vi "Get Element At (Dimensions).vi"(8 "error in (no error)":errorcluster, 10 "Index":i32[](array[numeric]), 11 "Array in":refnum<class "Array.lvclass">) -> (0 "error out":errorcluster, 2 "Element out":refnum<class "Data.lvclass">, 3 "Array out":refnum<class "Array.lvclass">)   [LabVIEW 2012, in "MDSplus.lvlib" / "Array.lvclass"]
doc: "Return a single element, if the passed number of dimension is equals to the dimension of dims field. Otherwise it returns the reshaped array corresponding to the passed dimension array. For example, if the array is bi-dimensional, a single dimension i will specify the i-th row.\nNote that this method may be implemented at this level since ArrayData has all the required information about data and dimension."
uses:
  <vilib>/MDSplus/Classes/Data_Class/Array_Class/Array.lvclass
  <vilib>/MDSplus/Classes/Data_Class/Data.lvclass
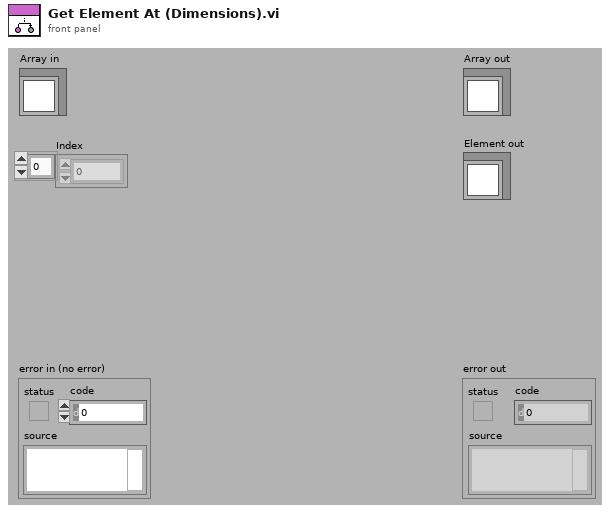
[diagram p1: front panel]
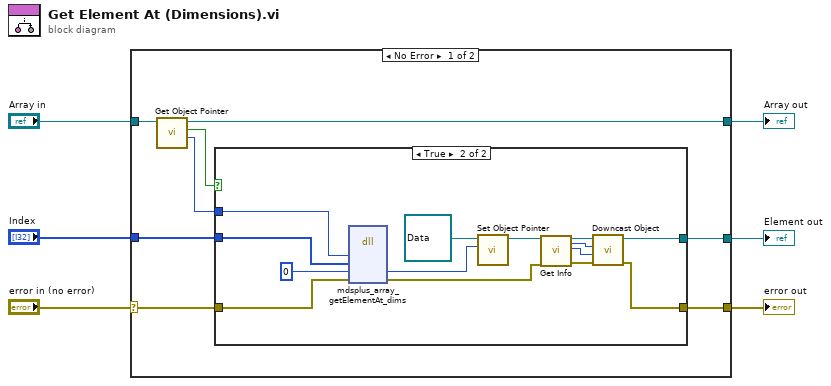
[diagram p0: block diagram]
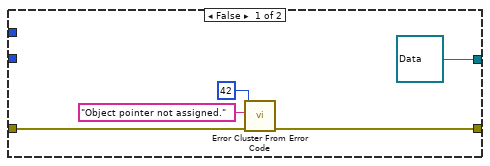
[diagram p2: hidden frame]
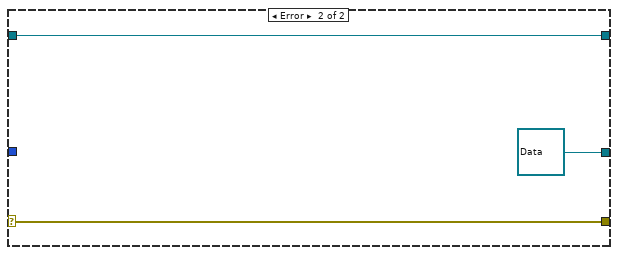
[diagram p3: hidden frame]
diagram:
  n1 = case shown="No Error" "error in (no error)" {
    selector: "error in (no error)" -> [w9 w36]
    tunnel: [w8 w36] -> w5
    tunnel: [w7 w35] -> w3
    tunnel: "Array in" -> [w12 w35]
    tunnel: "Index" -> [w14 _]
    tunnel: [w13 refnum<class "Data.lvclass"> refnum ("Data out")] -> w1
    frame No Error {
      n2 = call-dynamic "Get Object Pointer.vi"("Data in"=w12) -> ("Object Pointer"=w10:i64, "Assigned object pointer?"=w11:bool, "Data out"=w7:refnum<class "Array.lvclass">)  [unwired: 8 in]
      n3 = case shown="True" w11 {
        tunnel: w14 -> [_ w32]
        tunnel: [refnum<class "Data.lvclass"> refnum ("Data out") w24] -> w13
        tunnel: w10 -> [_ w23]
        tunnel: w9 -> [w16 w21]
        tunnel: [w15 w20] -> w8
        frame False {
          n4 = call <vilib>:"Error Cluster From Error Code.vi"("error in (no error)"=w16, "error message (\"\")"="Object pointer not assigned." ("error message (\"\")"), "error code (0)"=42) -> ("error out"=w15:errorcluster)  [unwired: 6 in]
        }
        frame True {
          n5 = dll-call lib="MDSobjectsLVShr" fn="mdsplus_array_getElementAt_dims"("lvArrayPtr"=w23, "lvIntArrHdlIn"=w32, "lvDataPtrOut"=i64 0, "error"=w21) -> ("lvDataPtrOut"=w30:i64, "error"=w22:errorcluster)  [unwired: 6 in, 2 out]
          n6 = call-dynamic "Set Object Pointer.vi"("Object Pointer"=w30, "Data in"=refnum<class "Data.lvclass"> refnum ("Data.lvclass")) -> ("Data out"=w29:refnum<class "Data.lvclass">)  [unwired: 9 in]
          n7 = call-dynamic "Get Info.vi"("Data in"=w29, "error in (no error)"=w22) -> ("Data out"=w28:refnum<class "Data.lvclass">, "Class type out"=w27:u8, "Data type out"=w26:u8, "error out"=w25:errorcluster)  [unwired: 12 in, 2 out]
          n8 = call <vilib>:"Downcast Object.vi"("error in (no error)"=w25, "Data Type"=w26, "Class Type"=w27, "Data in"=w28) -> ("error out"=w20:errorcluster, "Data out"=w24:refnum<class "Data.lvclass">)  [unwired: 6 in]
        }
      }
    }
    frame Error {
    }
  }
  "error out" <- w5
  "Array out" <- w3
  "Element out" <- w1
